vi "Find Location.vi"(3 "Make Vertical":bool, 4 "Wait Time":i32, 5 "Label":string, 6 "Side":T2=enum."right", 7 "Motion":enum16{"Joint", "Linear"}(ring), 8 "error in":errorcluster, 9 "Speed (mm/s)":dbl=50.0, 10 "Offset":T1 format="%.3f") -> (0 "error out":errorcluster)   [LabVIEW 2013]
uses:
  Prim/Fwd Kenimatics - array.vi
  <vilib>/Analysis/Matrix/NI_Matrix.lvlib
  <vilib>/Analysis/Matrix/Numeric/Multiply/Multiply - RM,RM.vi
  <vilib>/Analysis/Matrix/Datatypes/RealMatrix.ctl
  Goal.ctl
  ROS/Code/SubVIs/BaxterSide.ctl
panel:
  in  "Name":string
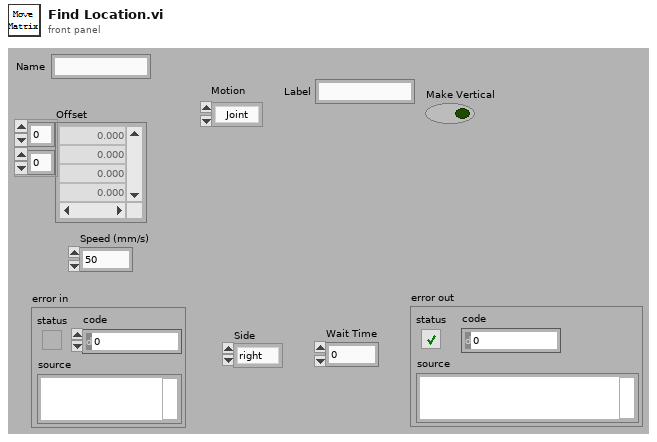
[diagram p1: front panel]
types:
  T1 = typedef "NI_Matrix.lvlib/RealMatrix.ctl" = dbl[][]
  T2 = typedef "BaxterSide.ctl" = enum16{"left", "right"}
  T3 = typedef "Goal.ctl" = cluster{"Segment":dbl, "T Matrix":T1, "Joints":dbl[], "Label":string, "Joint Motion":bool}
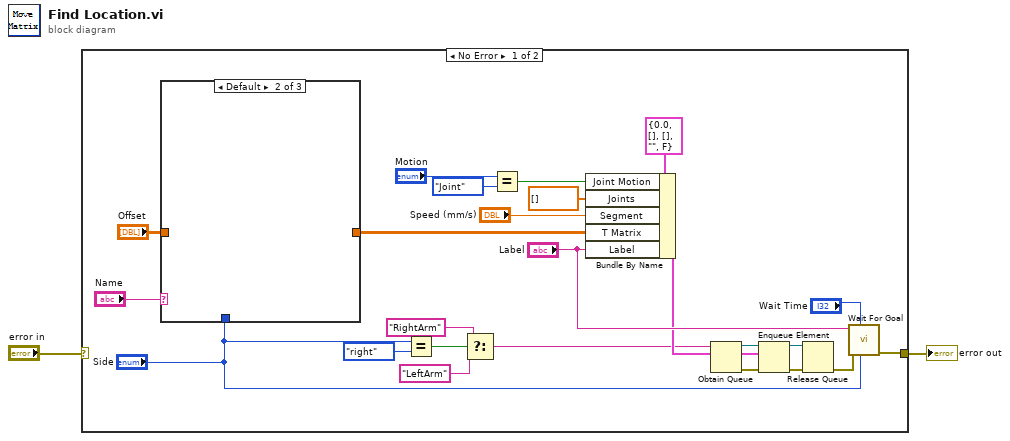
[diagram p0: block diagram]
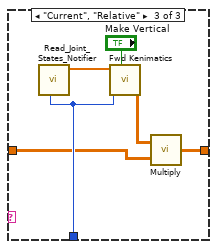
[diagram p3: hidden frame]
diagram:
  n1 = case shown="No Error" "error in" {
    selector: "error in" -> [_ w34]
    tunnel: [w17 w34] -> w1
    frame No Error {
      n2 = case shown="Default" "Name" {
        tunnel: "Offset" -> [w27 _ w30]
        tunnel: [w27 _ w28] -> w19
        tunnel: "Side" -> [_ _ w32]
        frame "Base", "World" {
        }
        frame Default {
        }
        frame "Current", "Relative" {
          n3 = call "Read_Joint_States_Notifier.vi"("Side"=w32) -> ("Positions"=w33:dbl[])  [unwired: 6 in, 1 out]
          n4 = call-poly "Fwd Kenimatics.vi"("Make Vertical"="Make Vertical", "Side"=w32, "Joints"=w33) -> ("Matrix"=w29:T1)  [unwired: 7 in, 1 out]
          n5 = call-poly <vilib>:"Multiply.vi"("Real Matrix B"=w30, "Real Matrix A"=w29) -> ("A * B"=w28:T1)
        }
      }
      n6 = Equal?(x="Side", y=BaxterSide."right") -> (x = y?=w8:bool)
      n7 = Select(t="RightArm" ("name (unnamed)"), s=w8, f="LeftArm") -> (s? t:f=w5:string)
      n8 = Equal?(x="Motion", y=enum16{"Joint", "Linear"}."Joint") -> (x = y?=w24:bool)
      n9 = Bundle By Name(cluster=T3 {"Segment"=0.0, "T Matrix"=[], "Joints"=[], "Label"="", "Joint Motion"=FALSE} ("Goal"), "Joint Motion"=w24, "Joints"=dbl[] [], "Segment"="Speed (mm/s)", "T Matrix"=w19, "Label"="Label") -> (w10:T3)
      n10 = Obtain Queue(name (unnamed)=w5, element data type=w10) -> (queue out=w14:refnum<queue>, error out=w13:errorcluster)  [unwired: 3 in, 1 out]
      n11 = Enqueue Element(queue=w14, element=w10, error in (no error)=w13) -> (queue out=w15:refnum<queue>, error out=w12:errorcluster)  [unwired: 1 in, 1 out]
      n12 = Release Queue(queue=w15, error in (no error)=w12) -> (error out=w11:errorcluster)  [unwired: 1 in, 2 out]
      n13 = call "Wait For Goal.vi"("Side"="Side", "wait time"="Wait Time", "error in"=w11, "Label"="Label") -> ("error out"=w17:errorcluster)  [unwired: 6 in, 1 out]
    }
    frame Error {
    }
  }
  "error out" <- w1
